vi "array1.vi"() -> ()   [LabVIEW 2020]
panel:
  out "text":string
  out "SDI":u8[](array[numeric]) format="%.0x"
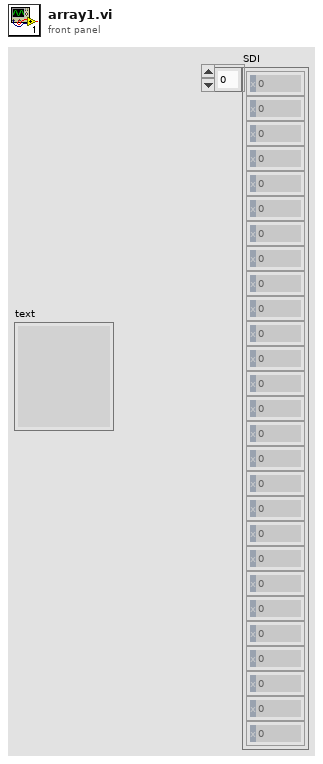
[diagram p1: front panel]
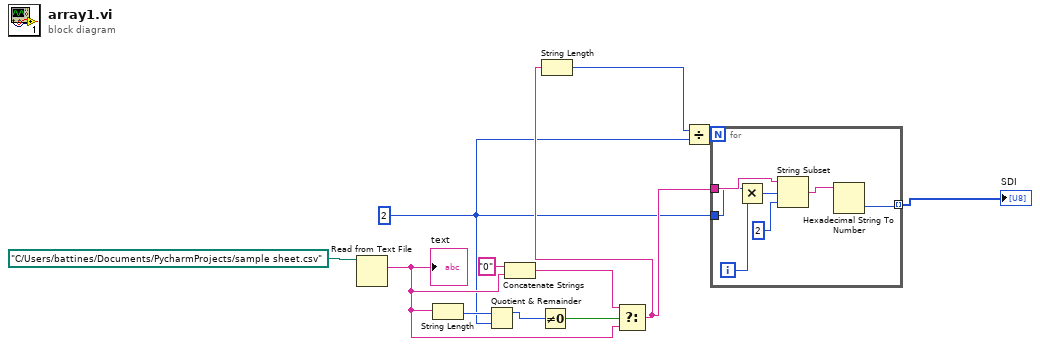
[diagram p0: block diagram]
diagram:
  w2 = 2 ("x")
  n1 = Read from Text File(file (use dialog)=path "C:/Users/battines/Documents/PycharmProjects/sample sheet.csv") -> (text=w6:string)  [unwired: 3 in, 3 out]
  "text" <- w6
  n2 = String Length(string=w6) -> (length=w10:i32)
  n3 = Quotient & Remainder(x=w10, y=w2) -> (x-y*floor(x/y)=w9:i32)  [unwired: 1 out]
  n4 = Concatenate Strings("0" ("string"), w6) -> (w7:string)
  n5 = Not Equal To 0?(x=w9) -> (x != 0?=w8:bool)
  n6 = Select(t=w7, s=w8, f=w6) -> (s? t:f=w3:string)
  n7 = String Length(string=w3) -> (length=w4:i32)
  n8 = Divide(x=w4, y=w2) -> (x/y=w5:dbl)
  n9 = for {
    N: w5 -> [_]
    tunnel: w3 -> [w15]
    tunnel: [w16] -> w1 mode=indexing
    tunnel: w2 -> [w14]
    i -> [w18]
    n10 = Multiply(x=w14, y=w18) -> (x*y=w19:i32)
    n11 = String Subset(string=w15, offset (0)=w19, length (rest)=2 ("length (rest)")) -> (substring=w17:string)
    n12 = Hexadecimal String To Number(string=w17) -> (number=w16:u32)  [unwired: 2 in, 1 out]
  }
  "SDI" <- w1
